vi "Write Directory.vi"(8 "error in (no error)":errorcluster, 10 "Path":path, 11 "TreeDirectory in":refnum<class "TreeDirectory.lvclass">) -> (0 "error out":errorcluster, 3 "TreeDirectory out":refnum<class "TreeDirectory.lvclass">)   [LabVIEW 2015, in "TreeDirectory.lvclass"]
doc: "This property gets or sets the Directory. The tree will query the path and will be populated with the contents of the directory on the writting call to this property.\n<b> </b> <b> </b>\n©2016 Q Software Innovations, LLC (QSI)\nwritten by Quentin Alldredge\nproduced in LabVIEW 2015\n\nsupport@qsoftwareinnovations.com\nwww.qsoftwareinnovations.com\n\nAll rights reserved.\n\nRedistribution and use in source and binary forms, with or without modification, are permitted provided that the following conditions are met:\n\n * Redistributions of source code must retain the above copyright notice, this list of conditions and the following disclaimer.\n * Redistributions in binary form must reproduce the above copyright notice, this list of conditions and the following disclaimer in the documentation and/or other materials provided with the distribution.\n * Neither the name of Q Software Innovations, LLC. nor the names of its contributors may be used to endorse or promote products derived from this software without specific prior written permission.\n\nTHIS SOFTWARE IS PROVIDED BY THE COPYRIGHT HOLDERS AND CONTRIBUTORS \"AS IS\" AND ANY EXPRESS OR IMPLIED WARRANTIES, INCLUDING, BUT NOT LIMITED TO, THE IMPLIED WARRANTIES OF MERCHANTABILITY AND FITNESS FOR A PARTICULAR PURPOSE ARE DISCLAIMED. IN NO EVENT SHALL THE COPYRIGHT OWNER OR CONTRIBUTORS BE LIABLE FOR ANY DIRECT, INDIRECT, INCIDENTAL, SPECIAL, EXEMPLARY, OR CONSEQUENTIAL DAMAGES (INCLUDING, BUT NOT LIMITED TO, PROCUREMENT OF SUBSTITUTE GOODS OR SERVICES; LOSS OF USE, DATA, OR PROFITS; OR BUSINESS INTERRUPTION) HOWEVER CAUSED AND ON ANY THEORY OF LIABILITY, WHETHER IN CONTRACT, STRICT LIABILITY, OR TORT (INCLUDING NEGLIGENCE OR OTHERWISE) ARISING IN ANY WAY OUT OF THE USE OF THIS SOFTWARE, EVEN IF ADVISED OF THE POSSIBILITY OF SUCH DAMAGE."
uses:
  TreeDirectory.lvclass
  TreeControl/TreeControl.lvclass
  TreeControl/Add Item Info Cluster.ctl
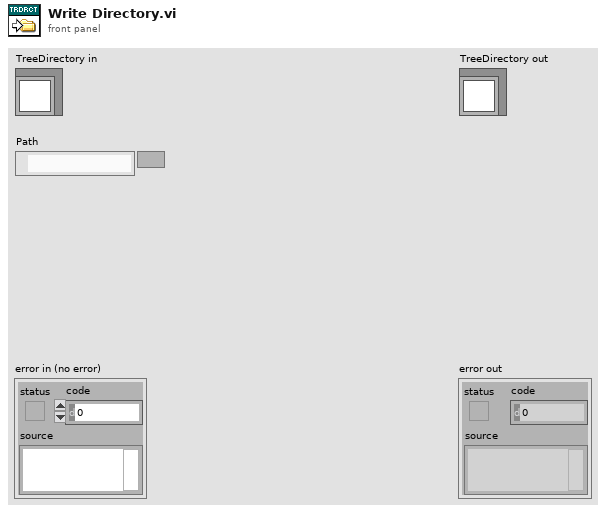
[diagram p1: front panel]
types:
  T1 = typedef "TreeControl.lvclass/Add Item Info Cluster.ctl" = cluster{"Parent Tag (\"\")":string, "Child Position (-1=End)":i32, "Left Cell String (\"\" = Same as Child Tag)":string, "Child Text[]":string[], "Child Tag":string, "Child Only? (F)":bool}
  T2 = typedef "imagedata.ctl" = cluster{"image type":i32, "image depth":i32, "image":u8[], "mask":u8[], "colors":u32[], "Rectangle":cluster{"left":i16, "top":i16, "right":i16, "bottom":i16}}
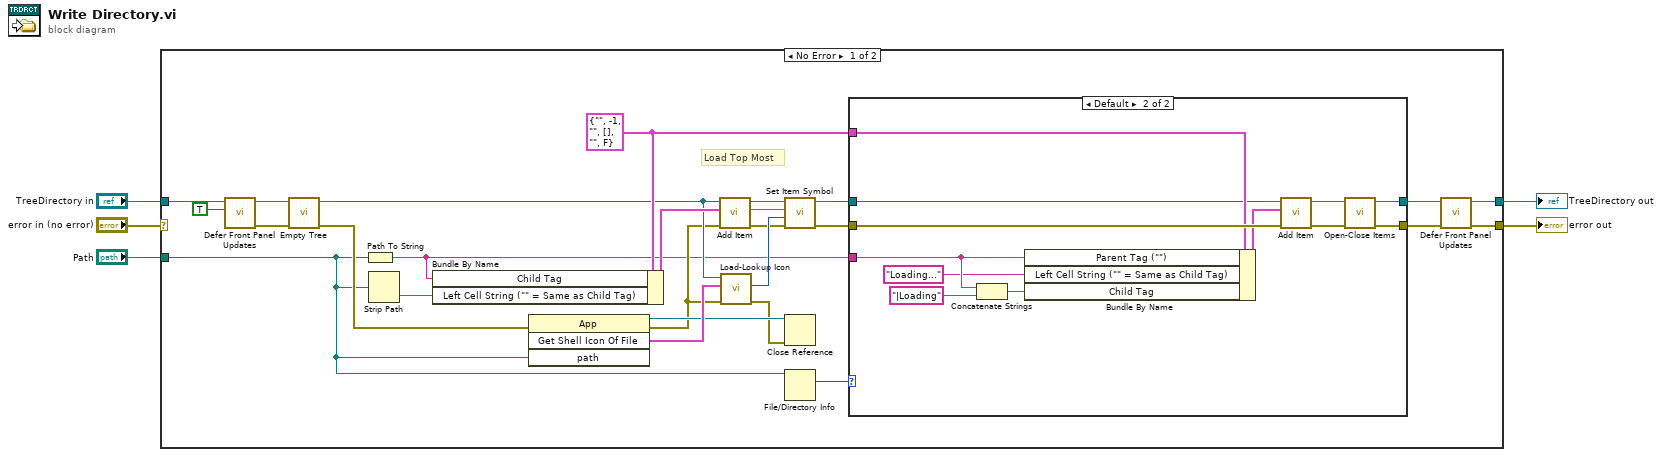
[diagram p0: block diagram]
diagram:
  n1 = case shown="No Error" "error in (no error)" {
    selector: "error in (no error)" -> [_ w47]
    tunnel: [w30 w47] -> w4
    tunnel: [w29 w46] -> w2
    tunnel: "TreeDirectory in" -> [w31 w46]
    tunnel: "Path" -> [w7 _]
    frame No Error {
      w19 = T1 {"Parent Tag (\"\")"="", "Child Position (-1=End)"=-1, "Left Cell String (\"\" = Same as Child Tag)"="", "Child Text[]"=[], "Child Tag"="", "Child Only? (F)"=FALSE} ("ItemInfo")
      # "Load Top Most"
      n2 = call "Defer Front Panel Updates.vi"("Defer Panel Updates (F)"=TRUE, "Tree in"=w31) -> ("error out"=w24:errorcluster, "Tree (dup)"=w25:refnum<class "TreeDirectory.lvclass">)  [unwired: 8 in]
      n3 = call "Empty Tree.vi"("error in (no error)"=w24, "Tree in"=w25) -> ("error out"=w10:errorcluster, "Tree (dup)"=w16:refnum<class "TreeDirectory.lvclass">)  [unwired: 8 in]
      n4 = Path To String(path=w7) -> (string=w8:string)
      n5 = Strip Path(path=w7) -> (name=w21:string)  [unwired: 1 out]
      n6 = Bundle By Name(cluster=w19, "Child Tag"=w8, "Left Cell String (\"\" = Same as Child Tag)"=w21) -> (w20:T1)
      n7 = invoke class="App" method="Get Shell Icon Of File"(error in=w10, "path"=w7) -> (reference out=w13:refnum<vi>, error out=w9:errorcluster, "GetShellIconOfFile"=w17:T2)  [unwired: 2 in, 1 out]
      n8 = call-dynamic "Add Item.vi"("error in (no error)"=w9, "ItemInfo"=w20, "Tree in"=w16) -> ("error out"=w14:errorcluster, "Add Item Tag"=w27:string, "Tree (dup)"=w15:refnum<class "TreeDirectory.lvclass">)  [unwired: 6 in]
      n9 = call "Load-Lookup Icon.vi"("error in (no error)"=w9, "Shell Icon"=w17, "TreeDirectory in"=w16) -> ("error out"=w11:errorcluster, "Icon Index"=w18:i32)  [unwired: 6 in, 1 out]
      n10 = call "Set Item Symbol.vi"("error in (no error)"=w14, "Symbol Index"=w18, "Tag"=w27, "Tree in"=w15) -> ("error out"=w28:errorcluster, "Tree (dup)"=w12:refnum<class "TreeDirectory.lvclass">)  [unwired: 6 in]
      n11 = Close Reference(reference=w13, error in (no error)=w11) -> ()  [unwired: 1 out]
      n12 = File/Directory Info(path=w7) -> (size=w6:i64)  [unwired: 1 in, 6 out]
      n13 = case shown="Default" w6 {
        tunnel: w28 -> [w32 w45]
        tunnel: [w33 w44] -> w23
        tunnel: [w32 w43] -> w22
        tunnel: w19 -> [_ w42]
        tunnel: w12 -> [w33 w40]
        tunnel: w8 -> [_ w38]
        frame 0 {
        }
        frame Default {
          n14 = Concatenate Strings(w38, "|Loading" ("string")) -> (w37:string)
          n15 = Bundle By Name(cluster=w42, "Parent Tag (\"\")"=w38, "Left Cell String (\"\" = Same as Child Tag)"="Loading..." ("string"), "Child Tag"=w37) -> (w41:T1)
          n16 = call-dynamic "Add Item.vi"("error in (no error)"=w45, "ItemInfo"=w41, "Tree in"=w40) -> ("error out"=w34:errorcluster, "Tree (dup)"=w35:refnum<class "TreeDirectory.lvclass">)  [unwired: 6 in, 1 out]
          n17 = call-dynamic "Open-Close Items.vi"("error in (no error)"=w34, "Tree in"=w35) -> ("error out"=w43:errorcluster, "Tree (dup)"=w44:refnum<class "TreeDirectory.lvclass">)  [unwired: 8 in]
        }
      }
      n18 = call "Defer Front Panel Updates.vi"("error in (no error)"=w22, "Tree in"=w23) -> ("error out"=w30:errorcluster, "Tree (dup)"=w29:refnum<class "TreeDirectory.lvclass">)  [unwired: 8 in]
    }
    frame Error {
    }
  }
  "error out" <- w4
  "TreeDirectory out" <- w2
